vi "QUBE-Servo 2 ROTPEN State-Space Model.vi"() -> ()   [LabVIEW 2016]
uses:
  <vilib>/imath/engines/lvmath2/RunTimeEngine/IndexRead/NIMS M(S,S).vi
  <instcachedir>/0/NIMS M(S,S)_AC51E74150A542F7991B9634C66F3096.lvgen/NIMS M(S,S)_AC51E74150A542F7991B9634C66F3096_000.vi
  <vilib>/imath/engines/lvmath2/RunTimeEngine/IndexRead/NIMS V(S).vi
  <instcachedir>/0/NIMS V(S)_0488751826AF41519A22953C041130DC.lvgen/NIMS V(S)_0488751826AF41519A22953C041130DC_000.vi
  <vilib>/imath/engines/lvmath2/RunTimeEngine/IndexReplace/NIMS M(S,S)=S.vi
  <instcachedir>/0/NIMS M(S,S)=S_98E40400474E4398B113AE20298B4F82.lvgen/NIMS M(S,S)=S_98E40400474E4398B113AE20298B4F82_000.vi
  <vilib>/imath/engines/lvmath2/RunTimeEngine/ErrorHandling/NIMS_Create Error From Enums.vi
  <vilib>/imath/engines/lvmath/Plug In/Control Design/BuiltInFunctions/ss/NIMS_CD_ss(A,B,C,D).vi
  <vilib>/imath/engines/lvmath2/RunTimeEngine/NodeEndStatement/NIMS_NodeEndStatement_Output.vi
  <instcachedir>/0/NIMS_NodeEndStatement_Output_53EC0D466D134D7ABD903AC30B43404B.lvgen/NIMS_NodeEndStatement_Output_53EC0D466D134D7ABD903AC30B43404B_010.vi
  <vilib>/imath/engines/lvmath2/RunTimeEngine/ErrorHandling/NIMS_Finalize Error.vi
  <vilib>/addons/Control Design/_Model Construction/Model File IO.llb/Model File IO Subvi/cd_Write Model to File (SS).vi
  <vilib>/addons/Control Design/_Utility/Model Viewer.llb/Model Viewer SubVI/cd_Draw State-Space Equation (SS).vi
  <vilib>/addons/Control Design/_Utility/NI_CD_Model Viewer.lvlib
  <vilib>/addons/Control Design/_Model Construction/NI_LinSys_Model File IO.lvlib
panel:
  out "Equation":picture
  in  "Motor Parameters":T1={"Rm (ohm)"=8.4, "km (V-s/rad)"=0.042, "kt (N-m/A)"=0.042} {"kt (N-m/A)" min=0.0 format="%_3g"; "km (V-s/rad)" min=0.0 format="%_3g"; "Rm (ohm)" min=0.0 format="%_3f"}
  in  "Model Name":string="qube_servo_2_rotpen_model"
  in  "Save Model":bool
  in  "Pendulum Parameters":T2={"Mp (kg)"=0.024, "Lr (m)"=0.085, "Lp (m)"=0.129, "Jr (kg.m^2)"=5.72e-05, "Dr (N.m.s/rad)"=0.0, "Jp (kg.m^2)"=3.33e-05, "Dp (N.m.s/rad)"=0.0, "g (m/s^2)"=9.81} {"g (m/s^2)" min=0.0 format="%_3g"; "Lr (m)" min=0.0 format="%_3g"; "Dr (N.m.s/rad)" min=0.0 format="%_3g"; "Jr (kg.m^2)" min=0.0 format="%_3g"; "Dp (N.m.s/rad)" min=0.0 format="%_3g"; "Jp (kg.m^2)" min=0.0 format="%_3g"; "Lp (m)" min=0.0 format="%_3g"; "Mp (kg)" min=0.0 format="%_3f"}
  in  "stop":bool
  # "Rotary Motion Platform"
  # "QUBE-Servo 2 | State-space Model"
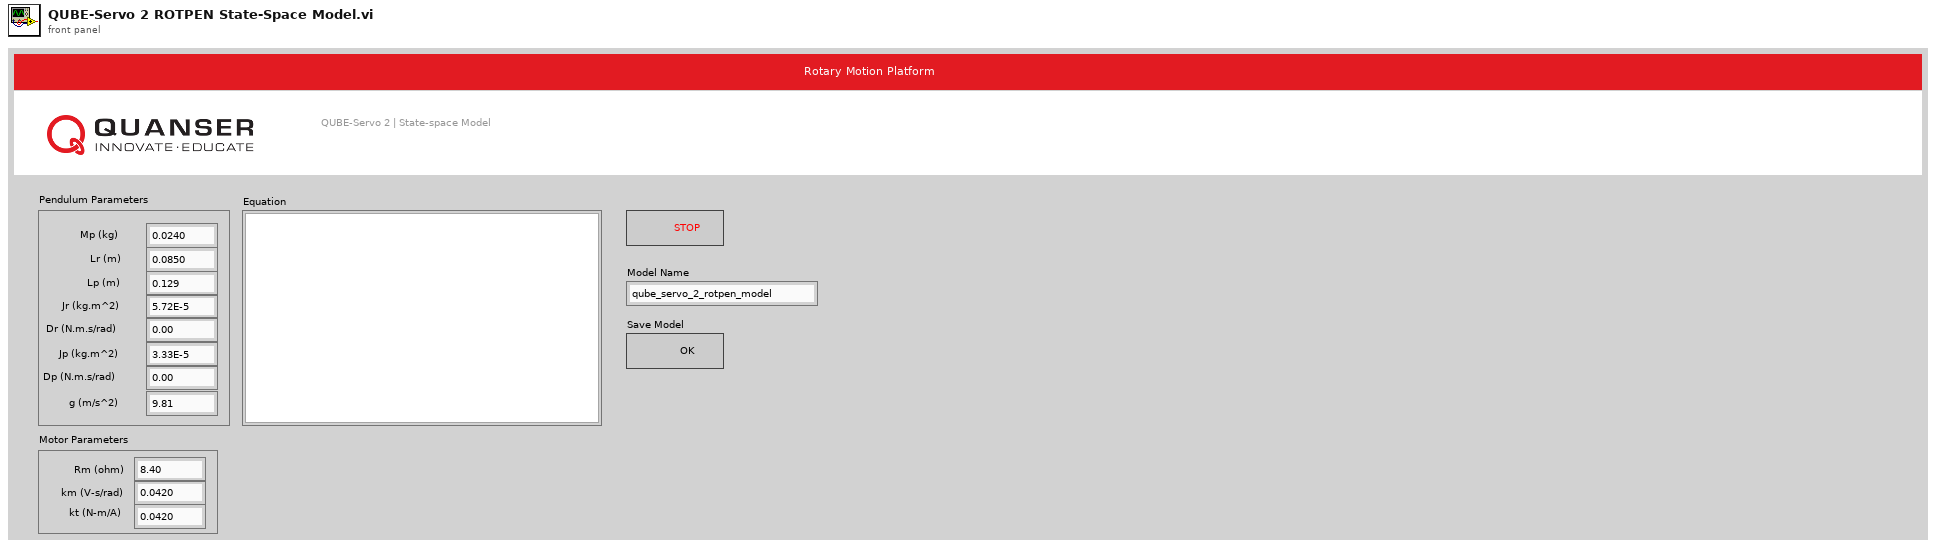
[diagram p1: front panel]
types:
  T1 = cluster{"Rm (ohm)":dbl, "km (V-s/rad)":dbl, "kt (N-m/A)":dbl}
  T2 = cluster{"Mp (kg)":dbl, "Lr (m)":dbl, "Lp (m)":dbl, "Jr (kg.m^2)":dbl, "Dr (N.m.s/rad)":dbl, "Jp (kg.m^2)":dbl, "Dp (N.m.s/rad)":dbl, "g (m/s^2)":dbl}
  T3 = typedef "NI_LinSys_Model Typedefs.lvlib/CD State Space Model (MIMO).ctl" = cluster{"properties":T4, "A":dbl[][], "B":dbl[][], "C":dbl[][], "D":dbl[][], "StateNames":string[], "Transport Delay":dbl[][]}
  T4 = typedef "NI_LinSys_Model Typedefs.lvlib/CD General Elements.ctl" = cluster{"Model name":string, "Input names":string[], "Output names":string[], "Input Delays":dbl[], "Output Delays":dbl[], "Sampling Time":dbl, "Notes":string}
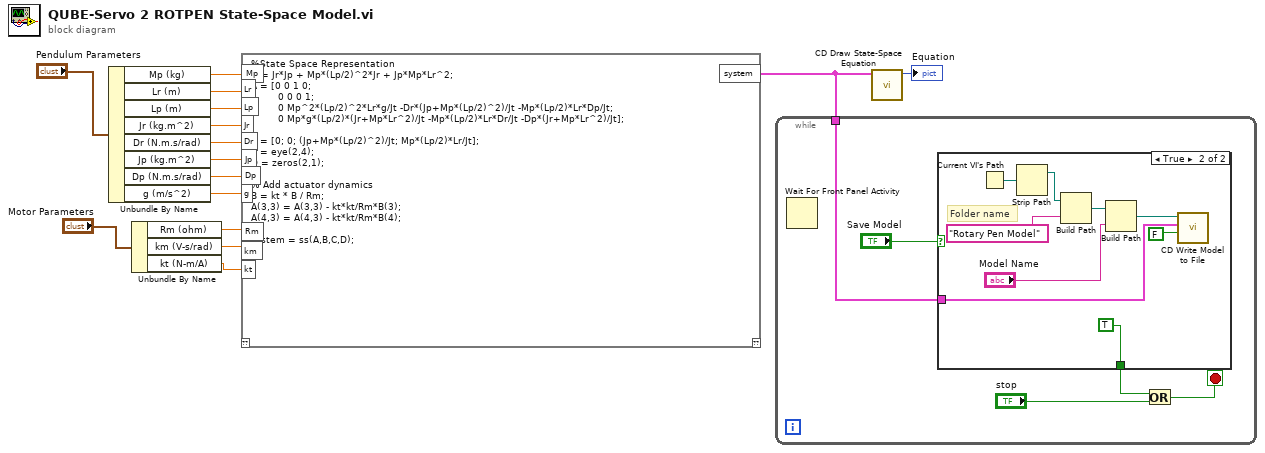
[diagram p0: block diagram]
diagram:
  n1 = Unbundle By Name("Pendulum Parameters") -> ("Mp (kg)"=w15:dbl, "Lr (m)"=w14:dbl, "Lp (m)"=w13:dbl, "Jr (kg.m^2)"=w12:dbl, "Dr (N.m.s/rad)"=w11:dbl, "Jp (kg.m^2)"=w10:dbl, "Dp (N.m.s/rad)"=w9:dbl, "g (m/s^2)"=w8:dbl)
  n2 = Unbundle By Name("Motor Parameters") -> ("Rm (ohm)"=w4:dbl, "km (V-s/rad)"=w3:dbl, "kt (N-m/A)"=w2:dbl)
  n3 = mathscript code="%State Space Representation\nJt = Jr*Jp + Mp*(Lp/2)^2*Jr + Jp*Mp*Lr^2;\nA = [0 0 1 0;\n         0 0 0 1;\n         0 Mp^2*(Lp/2)^2*Lr*g/Jt -Dr*(Jp+Mp*(Lp/2)^2)/Jt -Mp*(Lp/2)*Lr*Dp/Jt;\n         0 Mp*g*(Lp/2)*(Jr+Mp*Lr^2)/Jt -Mp*(Lp/2)*Lr*Dr/Jt -Dp*(Jr+Mp*Lr^2)/Jt];\n\nB = [0; 0; (Jp+Mp*(Lp/2)^2)/Jt; Mp*(Lp/2)*Lr/Jt];\nC = eye(2,4);\nD = zeros(2,1);\n\n% Add actuator dynamics\nB = kt * B / Rm;\nA(3,3) = A(3,3) - kt*kt/Rm*B(3);\nA(4,3) = A(4,3) - kt*kt/Rm*B(4);\n\nsystem = ss(A,B,C,D);"("Mp"=w15, "Lr"=w14, "Lp"=w13, "Jr"=w12, "Dr"=w11, "Jp"=w10, "Dp"=w9, "g"=w8, "kt"=w2, "km"=w3, "Rm"=w4) -> ("system"=w6:T3)  [unwired: 1 in, 1 out]
  n4 = while {
    tunnel: w6 -> [w16]
    stop <- w18 stop-if-true
    n5 = Wait For Front Panel Activity() -> ()  [unwired: 3 in, 1 out]
    n6 = case shown="True" "Save Model" {
      tunnel: w16 -> [_ w22]
      tunnel: [_ TRUE] -> w20
      frame False {
      }
      frame True {
        # "Folder name"
        n7 = Current VI's Path() -> (path=w23:path)
        n8 = Strip Path(path=w23) -> (stripped path=w27:path)  [unwired: 1 out]
        n9 = Build Path(base path=w27, name or relative path="Rotary Pen Model") -> (appended path=w28:path)
        n10 = Build Path(base path=w28, name or relative path="Model Name") -> (appended path=w25:path)
        n11 = call-poly <vilib>:"CD Write Model to File.vi"("Append to File? (new file:F)"=FALSE, "State-Space Model"=w22, "File Path (dialog if empty)"=w25) -> ()  [unwired: 6 in, 3 out]
      }
    }
    n12 = Or(x=w20, y="stop") -> (x .or. y?=w18:bool)
  }
  n13 = call-poly <vilib>:"CD Draw State-Space Equation.vi"("State-Space Model"=w6) -> ("Equation"=→"Equation":picture)  [unwired: 8 in, 2 out]
